vi "UDP Parse Packet Test.vi"() -> ()   [LabVIEW 2014, in "ESP8266 WiFi Wrapper.lvlib"]
uses:
  <vilib>/Aledyne-TSXperts/Arduino Compatible Compiler for LabVIEW/addons/ESP8266 WiFi Wrapper/ESP8266 WiFi Wrapper.lvlib
panel:
  out "Size of packet in bytes":i32
  out "Error Out":errorcluster
  in  "Error In":errorcluster
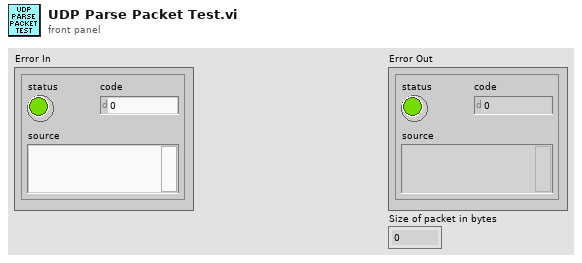
[diagram p1: front panel]
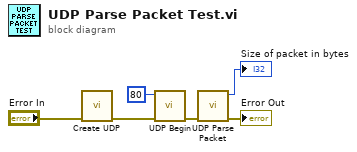
[diagram p0: block diagram]
diagram:
  n1 = call <vilib>:"Create UDP.vi"("Error In"="Error In") -> ("Error Out"=w4:errorcluster)  [unwired: 10 in]
  n2 = call <vilib>:"UDP Begin.vi"("Error In"=w4, "Port"=i16 80) -> ("Error Out"=w3:errorcluster)  [unwired: 8 in, 1 out]
  n3 = call <vilib>:"UDP Parse Packet.vi"("Error In"=w3) -> ("Error Out"=→"Error Out":errorcluster, "Size of packet in bytes"=→"Size of packet in bytes":i32)  [unwired: 9 in]
